vi "SaveDataAve.vi"(0 "Array":dbl[](array[numeric]), 1 "Save Data to File":bool) -> (3 "Current time (sec)":dbl format="%#_10g")   [LabVIEW 2018]
uses:
  Global 2.vi
  <vilib>/Utility/file.llb/Write To Spreadsheet File (DBL).vi
panel:
  out "Appended array":dbl[](array[numeric]) format="%#_10g"
  out "File name":string
  # "Saves data to spreadsheet file"
  # "Creates file with name including current time\nand header plus data"
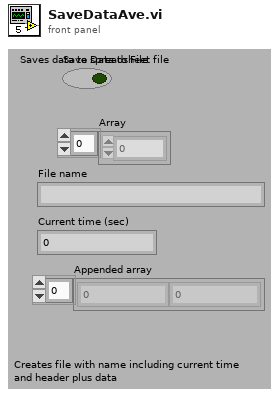
[diagram p1: front panel]
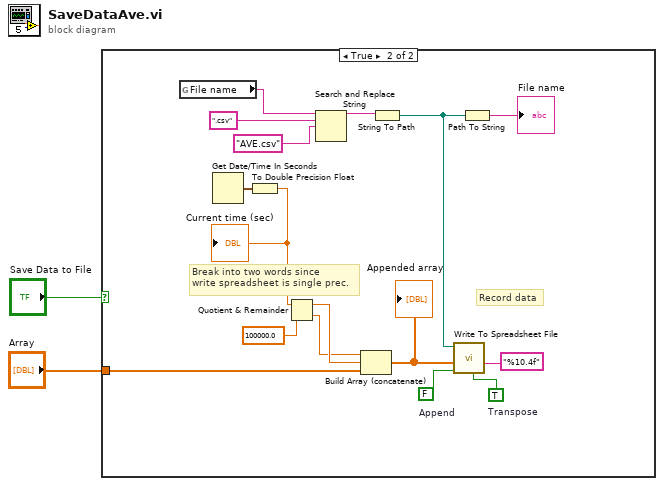
[diagram p0: block diagram]
diagram:
  n1 = case shown="True" "Save Data to File" {
    tunnel: "Array" -> [_ w16]
    frame False {
      # "Not writing file"
    }
    frame True {
      w14 = FALSE  # Append
      w15 = TRUE  # Transpose
      # "Record data"
      # "Break into two words since\nwrite spreadsheet is single prec."
      n2 = global read "Global 2.vi" "File name"() -> (w5:string)
      n3 = Get Date/Time In Seconds() -> (seconds since 1Jan1904=w12:timestamp)
      n4 = To Double Precision Float(number=w12) -> (double precision float=w7:dbl)
      "Current time (sec)" <- w7
      n5 = Quotient & Remainder(x=w7, y=100000.0) -> (x-y*floor(x/y)=w10:dbl, floor(x/y)=w8:dbl)
      n6 = Search and Replace String(input string=w5, search string=".csv", replace string="AVE.csv") -> (result string=w6:string)  [unwired: 5 in, 3 out]
      n7 = Build Array (concatenate) "Build Array"(w8, w10, w16) -> (w11:dbl[])
      "Appended array" <- w11
      n8 = String To Path(string=w6) -> (path=w17:path)
      n9 = call-poly <vilib>:"Write To Spreadsheet File.vi"("transpose? (no:F)"=w15, "format (%.3f)"="%10.4f", "append to file? (new file:F)"=w14, "1D data"=w11, "file path (dialog if empty)"=w17) -> ()  [unwired: 3 in, 1 out]
      n10 = Path To String(path=w17) -> (string=→"File name":string)
    }
  }
